vi "Start Data Logging Session.vi"(5 "Close Data Logging Specification Ref (T)":bool=TRUE, 7 "Data Logging Specification Ref in":T1, 8 "error in (no error)":errorcluster, 10 "Session Name in":string, 11 "Data Logging Manager Ref in":T2) -> (0 "error out":errorcluster, 2 "Session Name out":string, 3 "Data Logging Manager Ref out":T2)   [LabVIEW 2020, in "NI_VS Data Logging API.lvlib"]
doc: "Starts the data logging session specified by <B>Data Logging Specification in</B>. Use <B>Session Name in</B> to specify a unique name for the data logging session. You use this name to query and control logging operations during the logging session."
uses:
  <vilib>/NI VeriStand/Execution/DataLogging/NI_VS Data Logging API.lvlib
  <vilib>/NI VeriStand/Execution/DataLogging/IDataLogging Ref.ctl
  NationalInstruments.VeriStand.ClientAPI
  <vilib>/NI VeriStand/Execution/DataLogging/DataLoggingSpecification Ref.ctl
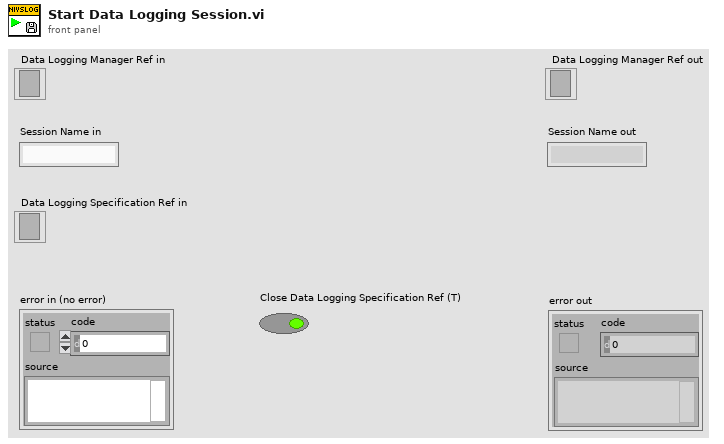
[diagram p1: front panel]
types:
  T1 = typedef "NI_VS Data Logging API.lvlib/DataLoggingSpecification Ref.ctl" = refnum<k24>
  T2 = typedef "NI_VS Data Logging API.lvlib/IDataLogging Ref.ctl" = refnum<k24>
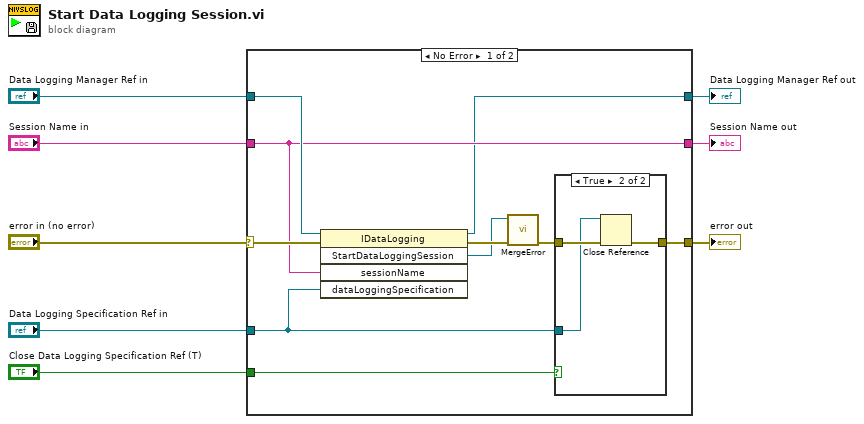
[diagram p0: block diagram]
diagram:
  n1 = case shown="No Error" "error in (no error)" {
    selector: "error in (no error)" -> [w18 w25]
    tunnel: [w9 w25] -> w7
    tunnel: [w13 w24] -> w6
    tunnel: "Data Logging Manager Ref in" -> [w17 w24]
    tunnel: [w16 w23] -> w4
    tunnel: "Session Name in" -> [w16 w23]
    tunnel: "Data Logging Specification Ref in" -> [w10 _]
    tunnel: "Close Data Logging Specification Ref (T)" -> [w11 _]
    frame No Error {
      n2 = invoke class="IDataLogging" method="StartDataLoggingSession"(reference=w17, error in=w18, "sessionName"=w16, "dataLoggingSpecification"=w10) -> (reference out=w13:T2, error out=w15:errorcluster, "StartDataLoggingSession"=w14:refnum<k24>)  [unwired: 1 in, 2 out]
      n3 = call <vilib>:"MergeError.vi"("error in (no error)"=w15, "Error"=w14) -> ("error out"=w12:errorcluster)  [unwired: 9 out]
      n4 = case shown="True" w11 {
        tunnel: w12 -> [w19 w22]
        tunnel: w10 -> [_ w21]
        tunnel: [w19 w20] -> w9
        frame False {
        }
        frame True {
          n5 = Close Reference(reference=w21, error in (no error)=w22) -> (error out=w20:errorcluster)
        }
      }
    }
    frame Error {
    }
  }
  "Data Logging Manager Ref out" <- w6
  "error out" <- w7
  "Session Name out" <- w4
